vi "Get-Keys-Section.vi"(8 "error in (no error)":errorcluster, 10 "Section":T1, 11 "Config in":refnum<class "Config.lvclass">) -> (0 "error out":errorcluster, 2 "Keys":string[](array[string]), 3 "Config out":refnum<class "Config.lvclass">)   [LabVIEW 2018, in "Config.lvclass"]
uses:
  Config.lvclass
  Delay Line/DelayLineLS4/LS4_parameters.ctl
  Config.lvclass/Config.ctl
  Delay Line/DelayLine.lvclass
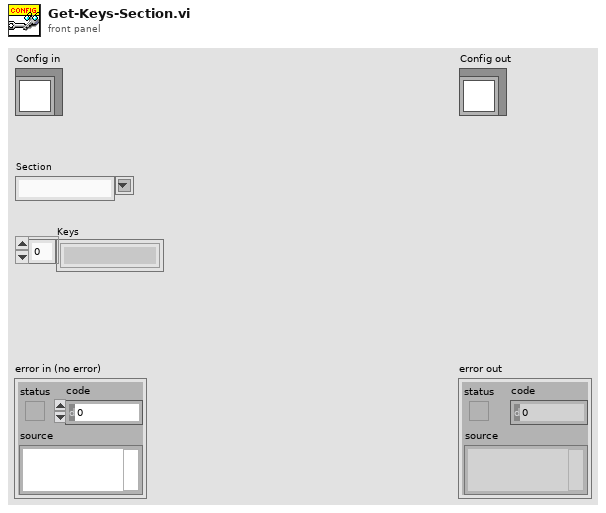
[diagram p1: front panel]
types:
  T1 = typedef "DelayLine.lvclass/LS4_parameters.ctl" = string
  T2 = cluster{"Keys":string[], "Keys-values":string[]}[]
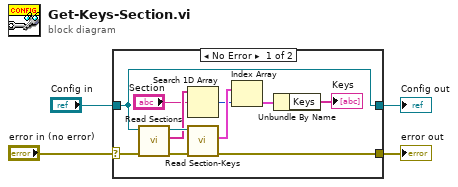
[diagram p0: block diagram]
diagram:
  n1 = case shown="No Error" "error in (no error)" {
    selector: "error in (no error)" -> [w14 w17]
    tunnel: [w12 w17] -> w3
    tunnel: [w15 w16] -> w1
    tunnel: "Config in" -> [w15 w16]
    frame No Error {
      n2 = call "Read Sections.vi"("error in (no error)"=w14, "Config in"=w15) -> ("error out"=w11:errorcluster, "Sections"=w7:string[], "Config out"=w13:refnum<class "Config.lvclass">)  [unwired: 7 in]
      n3 = Search 1D Array(1D array=w7, element="Section") -> (index of element=w5:i32)  [unwired: 1 in]
      n4 = call "Read Section-Keys.vi"("error in (no error)"=w11, "Config in"=w13) -> ("error out"=w12:errorcluster, "Section-Keys"=w10:T2)  [unwired: 7 in, 1 out]
      n5 = Index Array(array=w10, index=w5) -> (element=w9:cluster{"Keys":string[], "Keys-values":string[]})
      n6 = Unbundle By Name(w9) -> ("Keys"=→"Keys":string[])
    }
    frame Error {
    }
  }
  "error out" <- w3
  "Config out" <- w1
